vi "Test Triangle Class.vi"(8 "error in (no error)":errorcluster, 11 "TestCase in":refnum<class "Test FGEN.lvclass">) -> (0 "error out":errorcluster, 3 "TestCase out":refnum<class "Test FGEN.lvclass">)   [LabVIEW 2020, in "Test FGEN.lvclass"]
uses:
  Test FGEN.lvclass
  Libraries/FGen/Generador/Generador.lvclass
  Libraries/FGen/Generador/Generador.lvclass/Generador.ctl
  Libraries/FGen/Generador/Set signal type.vi
  <vilib>/addons/_JKI Toolkits/VI Tester/TestCase.llb/TestCase.lvclass
  C:/Program Files (x86)/National Instruments/LabVIEW 2020/vi.lib/addons/_JKI Toolkits/VI Tester/TestCase.llb/TestCase.lvclass
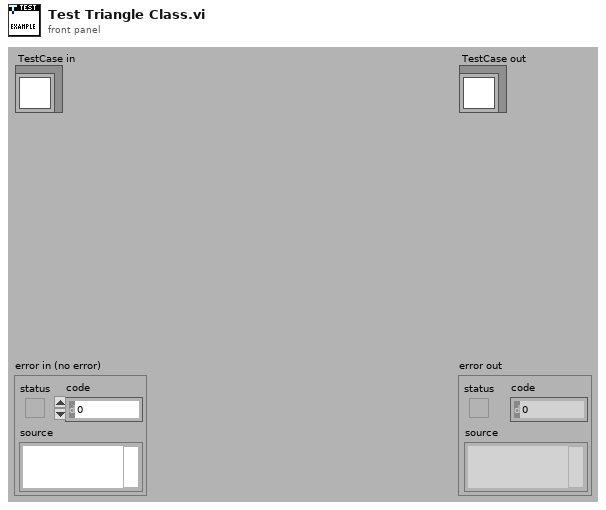
[diagram p1: front panel]
types:
  T1 = enum16{"Sine Wave", "Triangle Wave", "Square Wave", "Sawtooth Wave"}
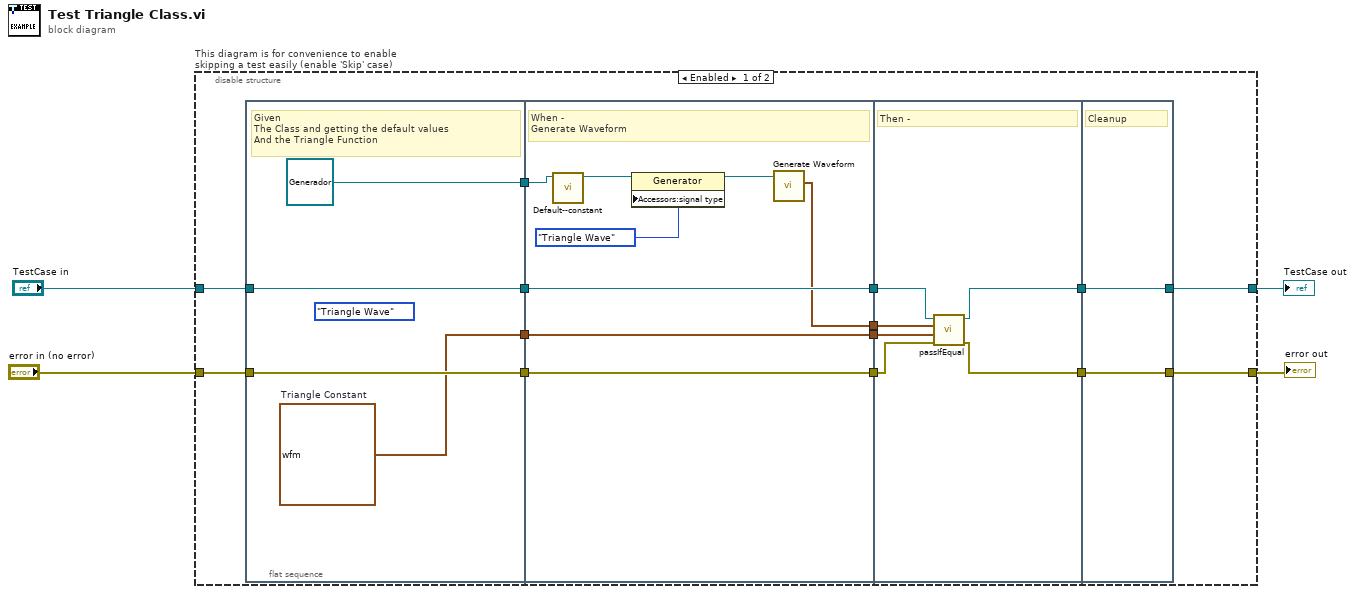
[diagram p0: block diagram]
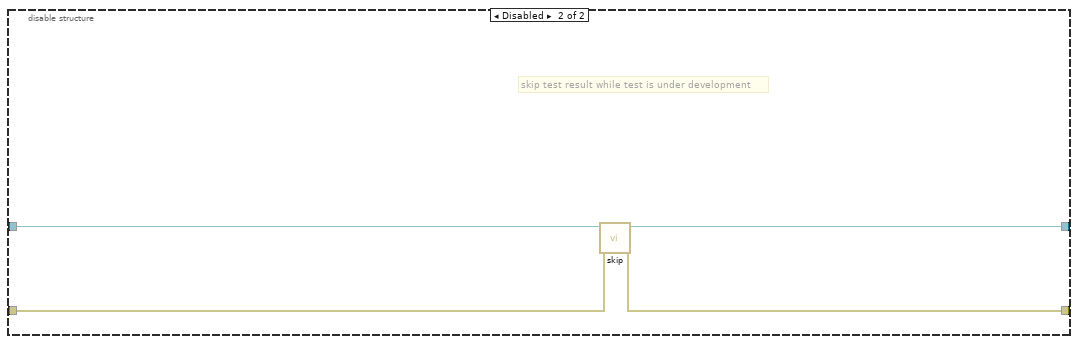
[diagram p2: hidden frame]
diagram:
  n1 = disable-structure "This diagram is for convenience to enable skipping a test easily (enable 'Skip' case)" shown="Enabled" {
    disable-tunnel: "TestCase in" -> [w14 w42]
    disable-tunnel: [w12 w40] -> w1
    disable-tunnel: [w13 w41] -> w3
    disable-tunnel: "error in (no error)" -> [w11 w39]
    frame Enabled {
      n2 = flat-sequence {
        tunnel: w14 -> [w22]
        tunnel: [w22] -> w18
        tunnel: w11 -> [w21]
        tunnel: [w21] -> w9
        tunnel: [w20] -> w7
        tunnel: [refnum<class "Generador.lvclass"> refnum ("FGen.lvlib:Generator")] -> w6
        tunnel: [w30] -> w17
        tunnel: w18 -> [w30]
        tunnel: [w29] -> w10
        tunnel: w9 -> [w29]
        tunnel: [w28] -> w8
        tunnel: w7 -> [w28]
        tunnel: w6 -> [w26]
        tunnel: [w23] -> w5
        tunnel: [w35] -> w16
        tunnel: [w34] -> w15
        tunnel: w17 -> [w36]
        tunnel: w10 -> [w33]
        tunnel: w8 -> [w32]
        tunnel: w5 -> [w31]
        tunnel: [w37] -> w13
        tunnel: [w38] -> w12
        tunnel: w16 -> [w38]
        tunnel: w15 -> [w37]
        frame #0 {
          (unwired) T1."Triangle Wave" ("signal type")
          w20 = waveform(dbl) {"t0"=timestamp(0 s since 1904-01-01), "dt"=0.001, "Y"=array[1000 elements]}  # Triangle Constant
          # "Given\nThe Class and getting the default values\nAnd the Triangle Function"
        }
        frame #1 {
          # "When -\nGenerate Waveform"
          n3 = call-dynamic "Default--constant.vi"("Generator in"=w26) -> ("Generator out"=w27:refnum<class "Generador.lvclass">)  [unwired: 9 in, 1 out]
          n4 = property class="Generator"(reference=w27, "Accessors:signal type"=T1."Triangle Wave" ("signal type")) -> (reference out=w25:refnum<class "Generador.lvclass">)  [unwired: 1 in, 1 out]
          n5 = call "Generate Waveform.vi"("Generator in"=w25) -> ("Waveform"=w23:waveform(dbl))  [unwired: 8 in, 2 out]
        }
        frame #2 {
          # "Then -"
          n6 = call-dynamic "passIfEqual.vi"("error in (no error)"=w33, "y"=w32, "x"=w31, "TestCase in"=w36) -> ("error out"=w34:errorcluster, "TestCase out"=w35:refnum<class "Test FGEN.lvclass">)  [unwired: 6 in]
        }
        frame #3 {
          # "Cleanup"
        }
      }
    }
    frame Disabled {
      # "skip test result while test is under development"
      n7 = call <vilib>:"skip.vi"("error in (no error)"=w39, "TestCase in"=w42) -> ("error out"=w41:errorcluster, "TestCase out"=w40:refnum<class "Test FGEN.lvclass">)  [unwired: 8 in]
    }
  }
  "error out" <- w3
  "TestCase out" <- w1
